vi "Get ctrl Primary Axis.vi"(3 "Controls":T1[](array[typedef])) -> (0 "Axes":dbl[](array[numeric]))   [LabVIEW 2014]
uses:
  TypeDefs/Axis Actions.ctl
  TypeDefs/SRE Enum.ctl
  Support Code/Robot Global Data.vi
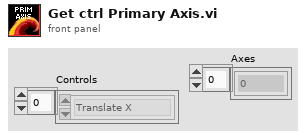
[diagram p1: front panel]
types:
  T1 = typedef "Axis Actions.ctl" = enum16{"Translate X", "Translate Y", "Rotate"}
  T2 = typedef "SRE Enum.ctl" = enum16{"Start", "Run", "End"}
  T3 = enum16{"X left ", "Y left", "Z left", "X right", "Y right", "Z right"}[]
  T4 = enum16{"X left ", "Y left", "Z left", "X right", "Y right", "Z right"}
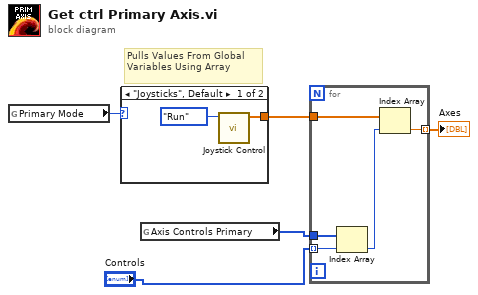
[diagram p0: block diagram]
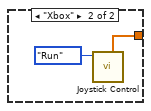
[diagram p2: hidden frame]
diagram:
  # "Pulls Values From Global Variables Using Array"
  n1 = global read "Robot Global Data.vi" "Primary Mode"() -> (w5:enum16{"Joysticks", "Xbox"})
  n2 = case shown="\"Joysticks\", Default" w5 {
    tunnel: [w6 w8] -> w4
    frame "Joysticks", Default {
      n3 = call "Joystick Control.vi"("Enum"=SRE_Enum."Run") -> ("Axis Output PJ"=w6:dbl[])  [unwired: 3 in, 5 out]
    }
    frame "Xbox" {
      n4 = call "Joystick Control.vi"("Enum"=SRE_Enum."Run") -> ("Axis Output PX"=w8:dbl[])  [unwired: 3 in, 5 out]
    }
  }
  n5 = global read "Robot Global Data.vi" "Axis Controls Primary"() -> (w2:T3)
  n6 = for {
    tunnel: "Controls" -> [w14] mode=indexing
    tunnel: [w13] -> w3 mode=indexing
    tunnel: w4 -> [w12]
    tunnel: w2 -> [w10]
    n7 = Index Array(array=w10, index=w14) -> (element=w11:T4)
    n8 = Index Array(array=w12, index=w11) -> (element=w13:dbl)
  }
  "Axes" <- w3
